vi "TranslateCoordinates.vi"(8 "X or Y":string, 11 "Graph Coord.":dbl) -> (3 "Pixel Coord.":i32)   [LabVIEW 2016, in "M1M3SupportEUI_Views.lvlib"]
uses:
  M1M3SupportEUI_Views.lvlib
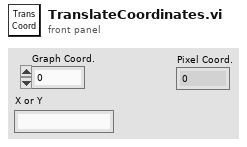
[diagram p1: front panel]
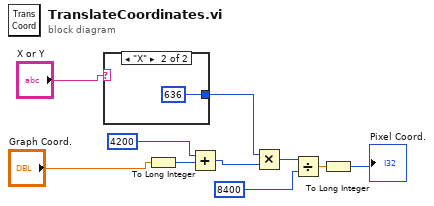
[diagram p0: block diagram]
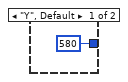
[diagram p2: hidden frame]
diagram:
  n1 = case shown="\"X\"" "X or Y" {
    tunnel: [580 ("x") 636 ("x")] -> w1
    frame "Y", Default {
    }
    frame "X" {
    }
  }
  n2 = To Long Integer(number="Graph Coord.") -> (32bit integer=w10:i32)
  n3 = Add(x=4200, y=w10) -> (x+y=w5:i32)
  n4 = Multiply(x=w1, y=w5) -> (x*y=w8:i32)
  n5 = Divide(x=w8, y=8400) -> (x/y=w4:dbl)
  n6 = To Long Integer(number=w4) -> (32bit integer=→"Pixel Coord.":i32)
